vi "4Pi Obj Lock - Crop Imag at Max.vi"(9 "edge size":i32=2, 11 "Input array":sgl[][](array[numeric])) -> (0 "Y":i32, 1 "X":i32, 2 "max value":sgl, 3 "subarray":sgl[][](array[numeric]))   [LabVIEW 2016]
panel:
  out "roi image":sgl[][](graph)
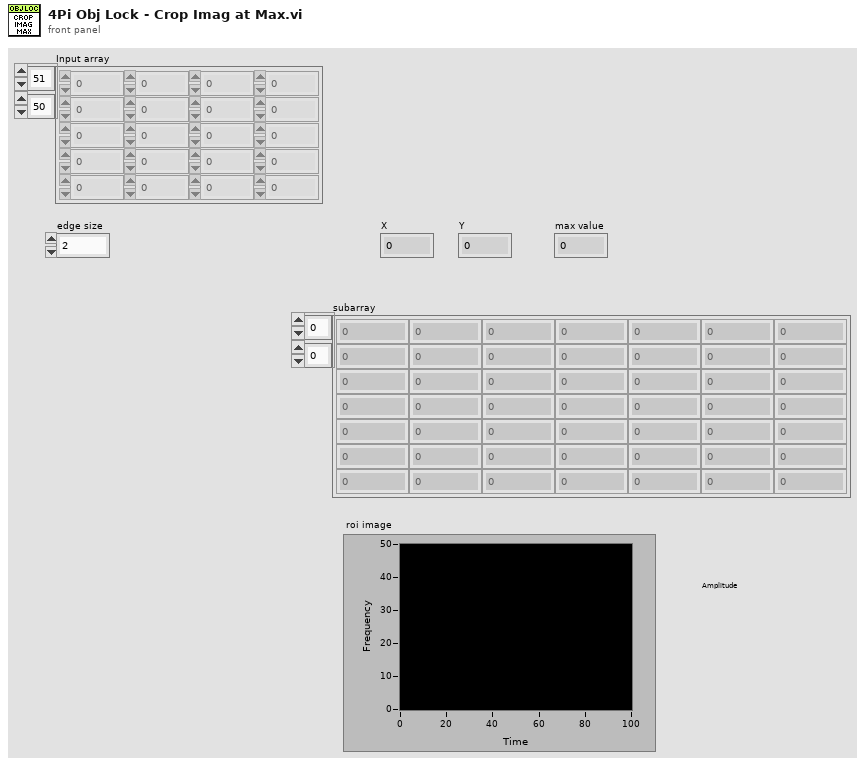
[diagram p1: front panel]
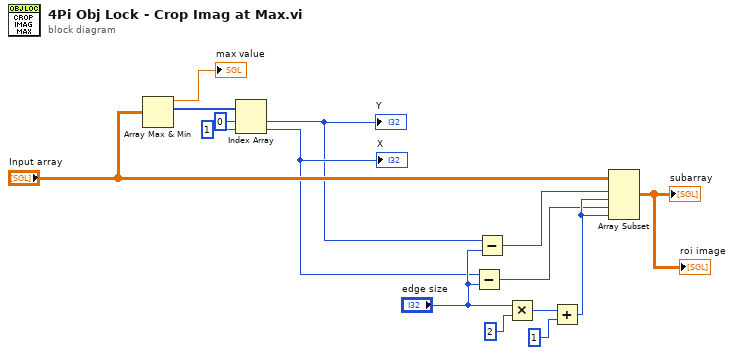
[diagram p0: block diagram]
diagram:
  n1 = Array Max & Min(array="Input array") -> (max value=→"max value":sgl, max index (indices)=w6:i32[])  [unwired: 2 out]
  n2 = Index Array(array=w6, index #1=0 ("index"), index #2=1 ("index")) -> (element #1=w2:i32, element #2=w3:i32)
  "X" <- w3
  "Y" <- w2
  n3 = Subtract(x=w3, y="edge size") -> (x-y=w9:i32)
  n4 = Subtract(x=w2, y="edge size") -> (x-y=w15:i32)
  n5 = Multiply(x="edge size", y=2) -> (x*y=w11:i32)
  n6 = Add(x=w11, y=1) -> (x+y=w13:i32)
  n7 = Array Subset(array="Input array", index (row)=w15, length (row)=w13, index (col)=w9, length (col)=w13) -> (→"subarray" →"roi image":sgl[][])
